vi "Initiate.vi"(8 "error in (no error)":errorcluster, 11 "Scope Instrument in":refnum<class "Scope Instrument.lvclass">) -> (0 "error out":errorcluster, 3 "Scope Instrument out":refnum<class "Scope Instrument.lvclass">)   [LabVIEW 2025, in "Scope.lvlib" / "Scope Instrument.lvclass"]
uses:
  Scope Instrument.lvclass
  Scope Instrument.lvclass/Scope Instrument.ctl
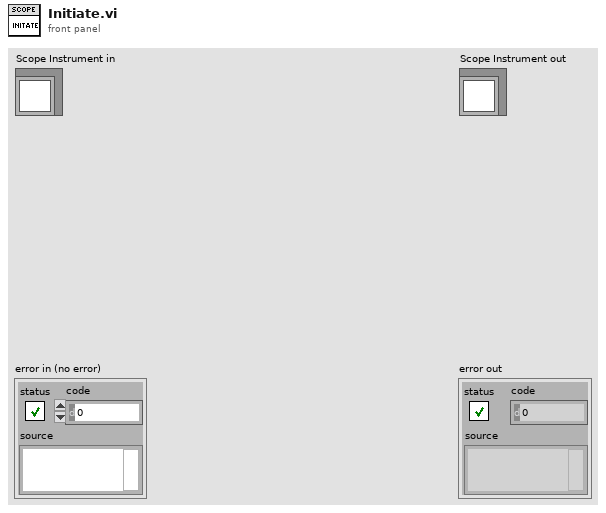
[diagram p1: front panel]
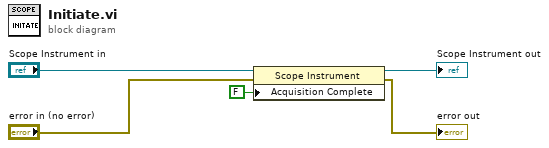
[diagram p0: block diagram]
diagram:
  n1 = property class="Scope Instrument"(reference="Scope Instrument in", error in="error in (no error)", "Acquisition Complete"=FALSE) -> (reference out=→"Scope Instrument out":refnum<class "Scope Instrument.lvclass">, error out=→"error out":errorcluster)
